vi "ProdaNG.TestValue.Del.vi"(8 "error in (no error)":errorcluster, 10 "TestStepId":i32, 11 "dbHandleIn":i32) -> (0 "error out":errorcluster, 3 "dbHandle":i32)   [LabVIEW 2016]
doc: "This function returns a product structure for a product, which is identified by a part and a serial number.\nImportant information: The field 'individual' was taken over from the field 'allgemein' of the legacy data directly. Because of this most products have the value 0 further on and only a few the value 1. \nParameter:\nhandle is an Integer, which is returned by the function Login() at the creation of a new connection.\nwabcoPartId is the Id of the part.\nserialNumber is the serial number of the product for the part above.\nproduct is a pointer on a product structure, which is filled if the returncode is 0. The structure must be defined in the calling program.\n\nReturncodes:\n0 No error\n< 0 ORACLE Error code\n6 (ERROR_INVALID_HANDLE) in case of an invalid handle\n1403 Record does not exist"
uses:
  prodllNG.dll
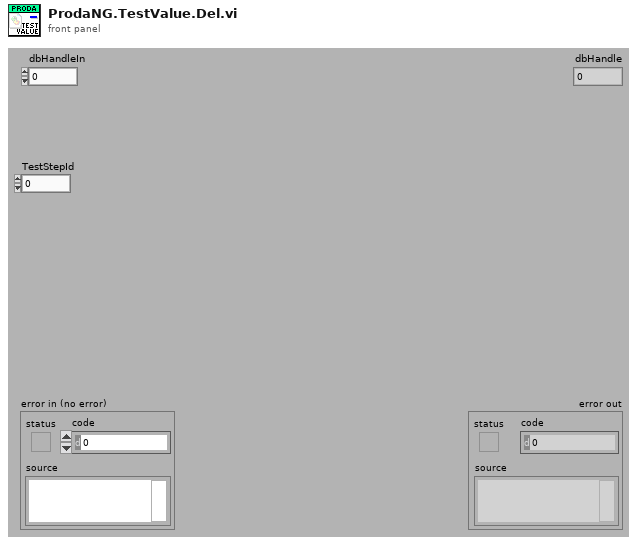
[diagram p1: front panel]
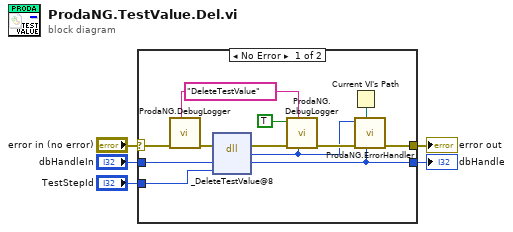
[diagram p0: block diagram]
diagram:
  n1 = case shown="No Error" "error in (no error)" {
    selector: "error in (no error)" -> [w12 w19]
    tunnel: [w17 w19] -> w4
    tunnel: "dbHandleIn" -> [w14 w18]
    tunnel: [w15 w18] -> w2
    tunnel: "TestStepId" -> [w6 _]
    frame No Error {
      w8 = "DeleteTestValue" ("cmd")
      n2 = call "ProdaNG.DebugLogger.vi"("cmd"=w8, "error in (no error)"=w12) -> ("error out"=w11:errorcluster)  [unwired: 9 in]
      n3 = dll-call lib="D:/Maszup/WABCO/SVN/LineTraceSystem/SOFTWARE/sources/Database/ProdaNG/prodllNG.dll" fn="_DeleteTestValue@8" ("ProDLL wrapper.dll:ProDLL_wrapper_GetWabcoParts_GetData")(error in=w11, "dbHandle"=w14, "testValueId"=w6) -> (error out=w10:errorcluster, "return type"=w7:i32, "dbHandle"=w15:i32)  [unwired: 3 in, 1 out]
      n4 = call "ProdaNG.DebugLogger.vi"("return type"=w7, "cmd"=w8, "error in (no error)"=w10, "done? (F)"=TRUE) -> ("error out"=w9:errorcluster)  [unwired: 7 in]
      n5 = Current VI's Path() -> (path=w16:path)
      n6 = call "ProdaNG.ErrorHandler.vi"("dbHandleIn"=w15, "Path"=w16, "error in"=w9, "output_parameter"=w7) -> ("error out"=w17:errorcluster)  [unwired: 7 in]
    }
    frame Error {
    }
  }
  "error out" <- w4
  "dbHandle" <- w2
